vi "publish status.vi"(8 "error in (no error)":errorcluster, 11 "Channel in":refnum<class "Channel.lvclass">) -> (0 "error out":errorcluster, 3 "Channel out":refnum<class "Channel.lvclass">)   [LabVIEW 2018, in "Channel.lvclass"]
uses:
  Channel.lvclass
  Channel.lvclass/Channel.ctl
  State Machine/State Machine.lvclass/State Machine.ctl
  State Machine/State Machine.lvclass
  Simulated_CCD_Camera/Simulated_CCD_Camera.lvclass
  RxTx/RxTx.lvclass
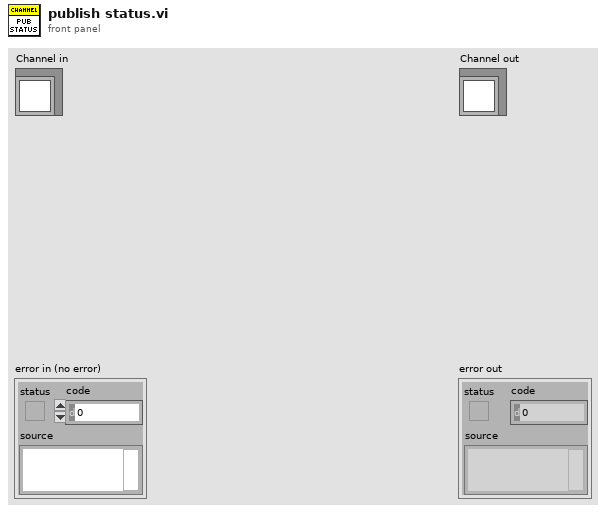
[diagram p1: front panel]
types:
  T1 = cluster{"CYCLES_DONE":u16, "LAST_IMAGE_NAME":string, "DISK_SPACE":u16, "FRAMES_DONE":u16, "CCD_STATUS":string, "CURRENT_TEMPERATURE":i16, "TEMPERATURE_STATUS":string, "FRAME_EXPOSURE_TIME":sgl, "ERROR":bool, "SERIAL_NUMBER":u16, "ACQUIRING":bool, "IMAGE_INDEX":u32, "SEQS_DONE":u16}
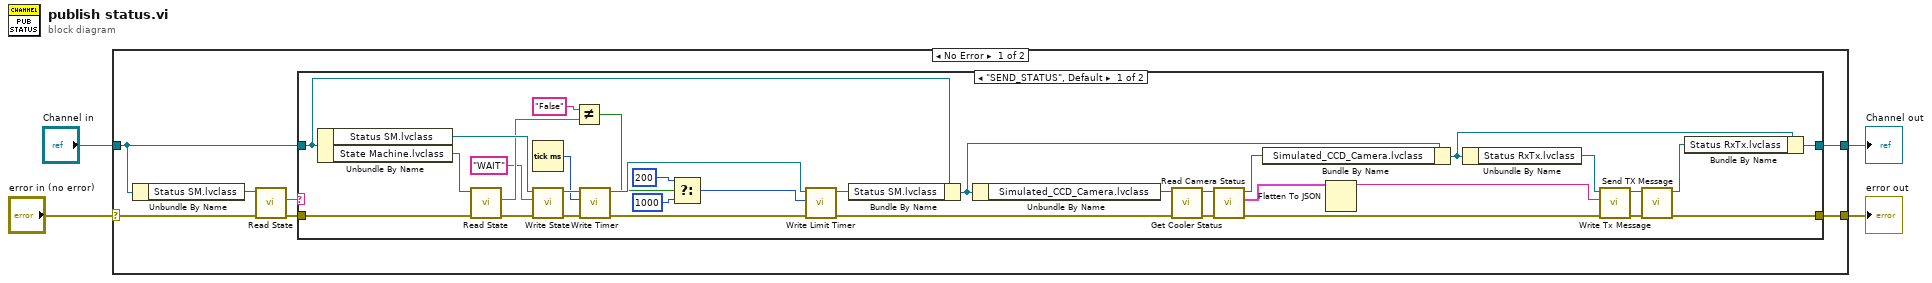
[diagram p0: block diagram]
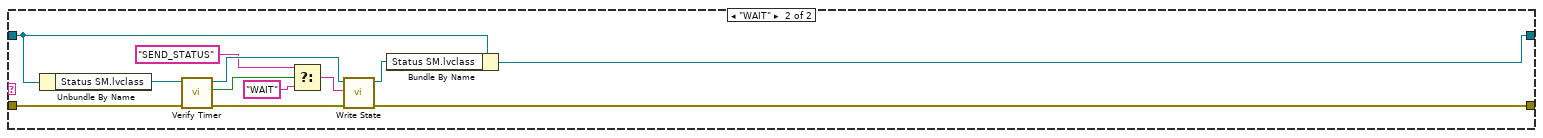
[diagram p2: hidden frame]
diagram:
  n1 = case shown="No Error" "error in (no error)" {
    selector: "error in (no error)" -> [w10 w59]
    tunnel: [w5 w59] -> w3
    tunnel: [w7 w58] -> w1
    tunnel: "Channel in" -> [w6 w58]
    frame No Error {
      n2 = Unbundle By Name(w6) -> ("Status SM.lvclass"=w11:refnum<class "State Machine.lvclass">)
      n3 = call-dynamic "Read State.vi"("error in (no error)"=w10, "State Machine in"=w11) -> ("error out"=w8:errorcluster, "State"=w9:string)  [unwired: 7 in, 1 out]
      n4 = case shown="\"SEND_STATUS\", Default" w9 {
        tunnel: w6 -> [w25 w56]
        tunnel: w8 -> [w26 w57]
        tunnel: [w20 w50] -> w5
        tunnel: [w21 w54] -> w7
        frame "SEND_STATUS", Default {
          n5 = Unbundle By Name(w25) -> ("Status SM.lvclass"=w34:refnum<class "State Machine.lvclass">, "State Machine.lvclass"=w35:refnum<class "State Machine.lvclass">)
          n6 = call-dynamic "Read State.vi"("error in (no error)"=w26, "State Machine in"=w35) -> ("error out"=w33:errorcluster, "State"=w32:string)  [unwired: 7 in, 1 out]
          n7 = Tick Count (ms)() -> (millisecond timer value=w39:u32)
          n8 = call-dynamic "Write State.vi"("error in (no error)"=w33, "State"="WAIT", "State Machine in"=w34) -> ("error out"=w40:errorcluster, "State Machine out"=w41:refnum<class "State Machine.lvclass">)  [unwired: 7 in]
          n9 = Not Equal?(x="False" ("State"), y=w32) -> (x != y?=w16:bool)
          n10 = call "Write Timer.vi"("error in (no error)"=w40, "Timer"=w39, "State Machine in"=w41) -> ("error out"=w36:errorcluster, "State Machine out"=w38:refnum<class "State Machine.lvclass">)  [unwired: 7 in]
          n11 = Select(t=200, s=w16, f=1000) -> (s? t:f=w31:i32)
          n12 = call "Write Limit Timer.vi"("error in (no error)"=w36, "Limit Timer"=w31, "State Machine in"=w38) -> ("error out"=w12:errorcluster, "State Machine out"=w37:refnum<class "State Machine.lvclass">)  [unwired: 7 in]
          n13 = Bundle By Name(cluster=w25, "Status SM.lvclass"=w37) -> (w45:refnum<class "Channel.lvclass">)
          n14 = Unbundle By Name(w45) -> ("Simulated_CCD_Camera.lvclass"=w15:refnum<class "Simulated_CCD_Camera.lvclass">)
          n15 = call-dynamic "Get Cooler Status.vi"("error in (no error)"=w12, "CCDCamera in"=w15) -> ("error out"=w13:errorcluster, "CCDCamera out"=w14:refnum<class "Simulated_CCD_Camera.lvclass">)  [unwired: 8 in]
          n16 = call "Read Camera Status.vi"("error in (no error)"=w13, "CCDCamera in"=w14) -> ("error out"=w42:errorcluster, "Camera Status"=w43:T1, "CCDCamera out"=w44:refnum<class "Simulated_CCD_Camera.lvclass">)  [unwired: 7 in]
          n17 = Bundle By Name(cluster=w45, "Simulated_CCD_Camera.lvclass"=w44) -> (w22:refnum<class "Channel.lvclass">)
          n18 = Flatten To JSON(anything=w43) -> (JSON string=w18:string)  [unwired: 2 in, 1 out]
          n19 = Unbundle By Name(w22) -> ("Status RxTx.lvclass"=w17:refnum<class "RxTx.lvclass">)
          n20 = call "Write Tx Message.vi"("error in (no error)"=w42, "Tx Message"=w18, "RxTx in"=w17) -> ("error out"=w19:errorcluster, "RxTx out"=w24:refnum<class "RxTx.lvclass">)  [unwired: 7 in]
          n21 = call "Send TX Message.vi"("error in (no error)"=w19, "RxTx in"=w24) -> ("error out"=w20:errorcluster, "RxTx out"=w23:refnum<class "RxTx.lvclass">)  [unwired: 8 in]
          n22 = Bundle By Name(cluster=w22, "Status RxTx.lvclass"=w23) -> (w21:refnum<class "Channel.lvclass">)
        }
        frame "WAIT" {
          n23 = Unbundle By Name(w56) -> ("Status SM.lvclass"=w55:refnum<class "State Machine.lvclass">)
          n24 = call "Verify Timer.vi"("error in (no error)"=w57, "State Machine in"=w55) -> ("error out"=w53:errorcluster, "time out"=w46:bool, "State Machine out"=w52:refnum<class "State Machine.lvclass">)  [unwired: 7 in]
          n25 = Select(t="SEND_STATUS", s=w46, f="WAIT") -> (s? t:f=w49:string)
          n26 = call-dynamic "Write State.vi"("error in (no error)"=w53, "State"=w49, "State Machine in"=w52) -> ("error out"=w50:errorcluster, "State Machine out"=w51:refnum<class "State Machine.lvclass">)  [unwired: 7 in]
          n27 = Bundle By Name(cluster=w56, "Status SM.lvclass"=w51) -> (w54:refnum<class "Channel.lvclass">)
        }
      }
    }
    frame Error {
    }
  }
  "error out" <- w3
  "Channel out" <- w1
